vi "Populate all INI Variables to Tree.vi"(8 "Error in":errorcluster caption="Error in (no error)", 9 "Include Value?":bool, 10 "Filter":string, 11 "TreeControl in":refnum<vi>) -> (0 "Error out":errorcluster)   [LabVIEW 2017, in "csm-iniViewer.lvlib"]
uses:
  csm-iniViewer.lvlib
  INI-Static-Variable-Support/INI-Static-Variable-Support.lvlib
  <userlib>/_NEVSTOP/Communicable State Machine(CSM)/addons/API-String-Arugments-Support/API String Arguments Support.lvlib
  <userlib>/_NEVSTOP/Communicable State Machine(CSM)/_tool/_ui/csm-ui-support.lvlib
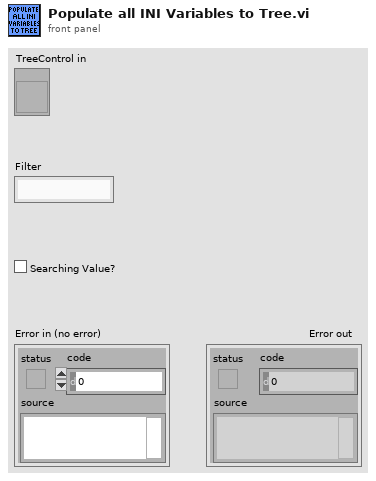
[diagram p1: front panel]
types:
  T1 = cluster{"Left Cell String":string, "Child Text":string[], "Child Tag":string, "Item Indent":i32, "Child Only?":bool, "Glyph Index":i32}[]
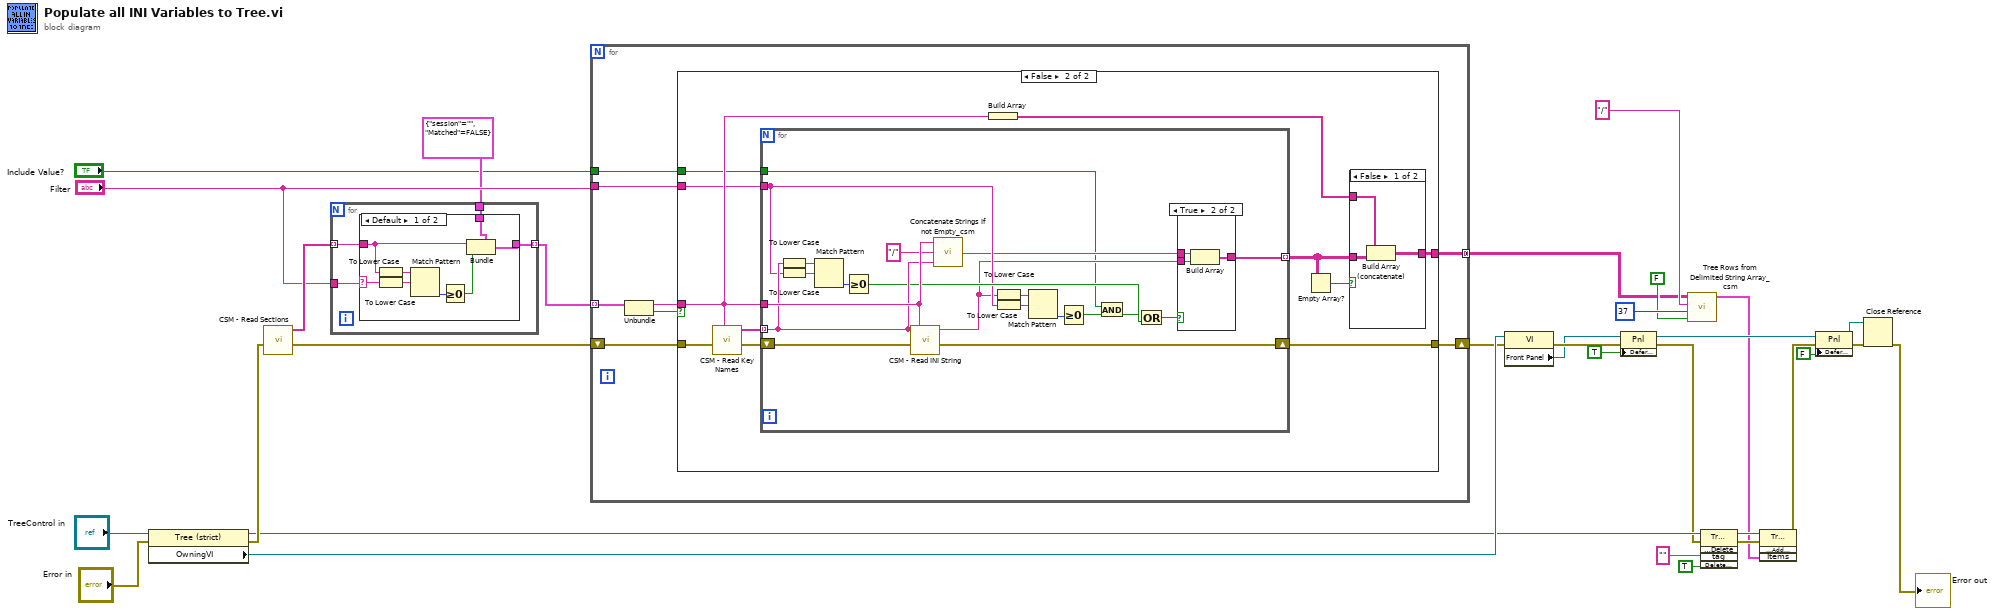
[diagram p0: block diagram]
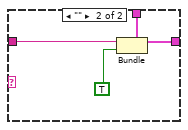
[diagram p2: hidden frame]
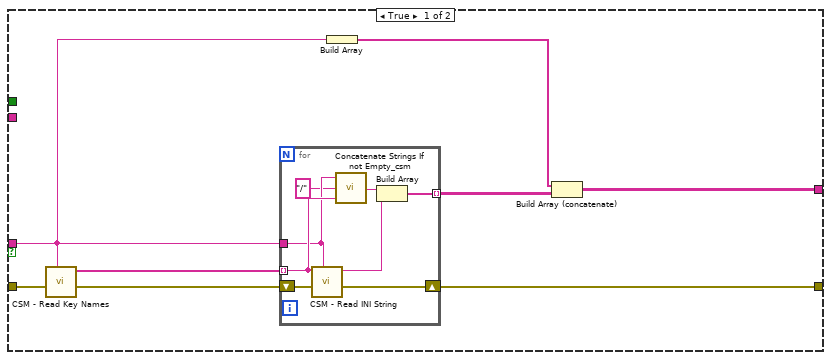
[diagram p3: hidden frame]
diagram:
  n1 = property class="Tree (strict)"(reference="TreeControl in", error in="Error in") -> (reference out=w29:refnum<vi>, error out=w31:errorcluster, "OwningVI"=w30:refnum<vi>)
  n2 = call "CSM - Read Sections.vi"("error in (no error)"=w31) -> ("error out"=w9:errorcluster, "Sections"=w5:string[])  [unwired: 7 in]
  n3 = for {
    tunnel: w5 -> [w34] mode=indexing
    tunnel: "Filter" -> [w35]
    tunnel: [w33] -> w3 mode=indexing
    tunnel: cluster{"session":string, "Matched":bool} {"session"="", "Matched"=FALSE} ("cluster") -> [w32]
    n4 = case shown="Default" w35 {
      selector: w35 -> [w43 _]
      tunnel: w34 -> [w39 w47]
      tunnel: [w40 w46] -> w33
      tunnel: w32 -> [w36 w44]
      frame Default {
        n5 = To Lower Case(string=w39) -> (all lower case string=w41:string)
        n6 = To Lower Case(string=w43) -> (all lower case string=w42:string)
        n7 = Match Pattern(string=w41, regular expression=w42) -> (offset past match=w38:i32)  [unwired: 1 in, 3 out]
        n8 = Greater Or Equal To 0?(x=w38) -> (x >= 0?=w37:bool)
        n9 = Bundle(cluster=w36, "session"=w39, "Matched"=w37) -> (w40:cluster{"session":string, "Matched":bool})
      }
      frame "" {
        n10 = Bundle(cluster=w44, "session"=w47, "Matched"=TRUE) -> (w46:cluster{"session":string, "Matched":bool})
      }
    }
  }
  n11 = for {
    tunnel: w3 -> [w52] mode=indexing
    shift-right: [w54] -> w20
    shift-left: w9 -> [w55]
    tunnel: [w53] -> w8 mode=concatenating
    tunnel: "Filter" -> [w49]
    tunnel: "Include Value?" -> [w48]
    n12 = Unbundle(w52) -> ("session"=w51:string, "Matched"=w50:bool)
    n13 = case shown="False" w50 {
      tunnel: w55 -> [w63 w82]
      tunnel: [w61 w80] -> w54
      tunnel: [w58 w78] -> w53
      tunnel: w51 -> [w56 w76]
      tunnel: w49 -> [_ w73]
      tunnel: w48 -> [_ w72]
      frame True {
        n14 = call "CSM - Read Key Names.vi"("Section Name (\"\" as Default)"=w56, "error in (no error)"=w63) -> ("error out"=w62:errorcluster, "Keys"=w60:string[])  [unwired: 6 in]
        n15 = for {
          tunnel: w56 -> [w68]
          tunnel: w60 -> [w69] mode=indexing
          shift-right: [w70] -> w61
          shift-left: w62 -> [w71]
          tunnel: [w65] -> w59 mode=indexing
          n16 = call "CSM - Read INI String.vi"("Section Name (\"\" as Default)"=w68, "error in (no error)"=w71, "Variable Name"=w69) -> ("error out"=w70:errorcluster, "Value"=w66:string)  [unwired: 4 in, 1 out]
          n17 = call <userlib>:"Concatenate Strings If not Empty_csm.vi"("String"=w69, "seperator(:)"="/", "prefix"=w68) -> ("result"=w67:string)  [unwired: 2 in]
          n18 = Build Array(w67, w66) -> (w65:string[])
        }
        n19 = Build Array(w56) -> (w57:string[])
        n20 = Build Array (concatenate)(w57, w59) -> (w58:string[][])
      }
      frame False {
        n21 = call "CSM - Read Key Names.vi"("Section Name (\"\" as Default)"=w76, "error in (no error)"=w82) -> ("error out"=w81:errorcluster, "Keys"=w79:string[])  [unwired: 6 in]
        n22 = for {
          tunnel: w76 -> [w103]
          tunnel: w79 -> [w98] mode=indexing
          shift-right: [w104] -> w80
          shift-left: w81 -> [w105]
          tunnel: [w102] -> w75 mode=indexing
          tunnel: w73 -> [w96]
          tunnel: w72 -> [w86]
          n23 = To Lower Case(string=w98) -> (all lower case string=w100:string)
          n24 = To Lower Case(string=w96) -> (all lower case string=w99:string)
          n25 = Match Pattern(string=w100, regular expression=w99) -> (offset past match=w101:i32)  [unwired: 1 in, 3 out]
          n26 = Greater Or Equal To 0?(x=w101) -> (x >= 0?=w97:bool)
          n27 = call "CSM - Read INI String.vi"("Section Name (\"\" as Default)"=w103, "error in (no error)"=w105, "Variable Name"=w98) -> ("error out"=w104:errorcluster, "Value"=w89:string)  [unwired: 4 in, 1 out]
          n28 = call <userlib>:"Concatenate Strings If not Empty_csm.vi"("String"=w98, "seperator(:)"="/", "prefix"=w103) -> ("result"=w95:string)  [unwired: 2 in]
          n29 = To Lower Case(string=w89) -> (all lower case string=w93:string)
          n30 = To Lower Case(string=w96) -> (all lower case string=w92:string)
          n31 = Match Pattern(string=w93, regular expression=w92) -> (offset past match=w91:i32)  [unwired: 1 in, 3 out]
          n32 = Greater Or Equal To 0?(x=w91) -> (x >= 0?=w90:bool)
          n33 = And(x=w86, y=w90) -> (x .and. y?=w87:bool)
          n34 = Or(x=w87, y=w97) -> (x .or. y?=w88:bool)
          n35 = case shown="True" w88 {
            tunnel: [_ w108] -> w102
            tunnel: w95 -> [_ w107]
            tunnel: w89 -> [_ w106]
            frame False {
            }
            frame True {
              n36 = Build Array(w107, w106) -> (w108:string[])
            }
          }
        }
        n37 = Build Array(w76) -> (w77:string[])
        n38 = Empty Array?(array=w75) -> (empty?=w74:bool)
        n39 = case shown="False" w74 {
          tunnel: [w85 _] -> w78
          tunnel: w77 -> [w84 _]
          tunnel: w75 -> [w83 _]
          frame False {
            n40 = Build Array (concatenate)(w84, w83) -> (w85:string[][])
          }
          frame True {
          }
        }
      }
    }
  }
  n41 = property class="VI"(reference=w30, error in=w20) -> (error out=w14:errorcluster, "Front Panel"=w13:refnum<vi>)  [unwired: 1 out]
  n42 = property class="Pnl"(reference=w13, error in=w14, "Defer Panel Updates"=TRUE) -> (reference out=w19:refnum<vi>, error out=w17:errorcluster)
  n43 = call <userlib>:"Tree Rows from Delimited String Array_csm.vi"("Use Child Only? (F)"=FALSE ("Use Child Only?"), "Default Symbol"=37, "Delimiter"="/", "Items (Delimited)"=w8) -> ("Item to Add[]"=w10:T1)  [unwired: 6 in, 1 out]
  n44 = invoke on="Invoke Node" class="Tree (strict)" method="Edit Tree Items.Delete"(reference=w29, error in=w17, "tag"="" ("Tag"), "Delete Children"=TRUE ("Delete Children?")) -> (reference out=w12:refnum<vi>, error out=w11:errorcluster)  [unwired: 1 in, 3 out]
  n45 = invoke on="Invoke Node" class="Tree (strict)" method="Edit Tree Items.Add Multiple Items to End"(reference=w12, error in=w11, "Items"=w10) -> (error out=w18:errorcluster)  [unwired: 1 in, 3 out]
  n46 = property class="Pnl"(reference=w19, error in=w18, "Defer Panel Updates"=FALSE) -> (reference out=w16:refnum<vi>, error out=w15:errorcluster)
  n47 = Close Reference(reference=w16, error in (no error)=w15) -> (error out=→"Error out":errorcluster)
